vi "Subset Status.vi"(8 "error in (no error)":errorcluster, 9 "count (1)":u64=1, 10 "index":u64, 11 "status pointer in":refnum<class "Status.lvclass">) -> (0 "error out":errorcluster, 1 "index + count":u64, 2 "subset status pointer":refnum<class "Status.lvclass">, 3 "status pointer out":refnum<class "Status.lvclass">)   [LabVIEW 2017, in "DSF Core.lvlib" / "Status.lvclass"]
uses:
  Status.lvclass
  C:/Git/DSF/LabVIEW-Memory/Source/Classes/Pointer/Pointer.lvclass
  LabVIEW-Memory/Source/Classes/Pointer/Pointer.lvclass
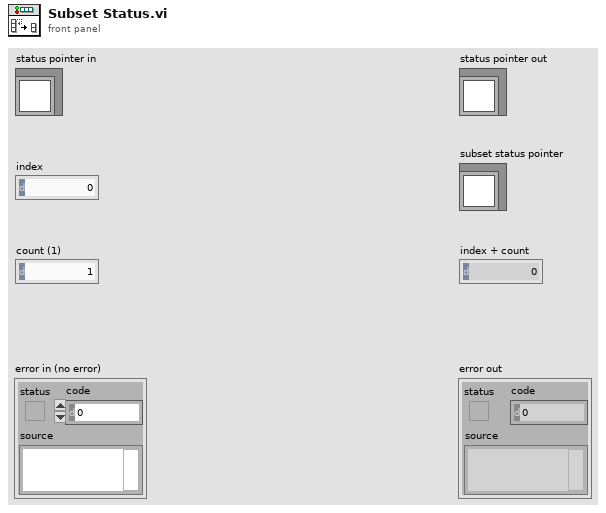
[diagram p1: front panel]
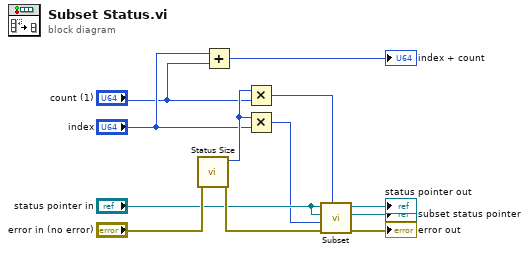
[diagram p0: block diagram]
diagram:
  n1 = call "Status Size.vi"("error in (no error)"="error in (no error)") -> ("error out"=w12:errorcluster, "size"=w5:u64)  [unwired: 9 in]
  n2 = Add(x="index", y="count (1)") -> (x+y=→"index + count":u64)
  n3 = Multiply(x=w5, y="count (1)") -> (x*y=w6:u64)
  n4 = Multiply(x=w5, y="index") -> (x*y=w4:u64)
  n5 = call "Subset.vi"("length (-1: rest)"=w6, "error in (no error)"=w12, "offset (0)"=w4, "subset Pointer type"="status pointer in", "base Pointer in"="status pointer in") -> ("error out"=→"error out":errorcluster, "subset Pointer"=→"subset status pointer":refnum<class "Status.lvclass">, "base Pointer out"=→"status pointer out":refnum<class "Status.lvclass">)  [unwired: 3 in, 1 out]
